vi "Initialize.vi"(8 "error in":errorcluster, 10 "parameters":variant, 11 "Sync Channel in":refnum<class "Synchronization Channel.lvclass">) -> (0 "error out":errorcluster, 2 "summary":T2[](array[typedef]), 3 "data value reference":T1)   [LabVIEW 2025, in "Synchronization.lvlib" / "Synchronization Channel.lvclass"]
doc: "This Vi initializes the data of a node its default state.\nThe object is not created inside of this ViI, beacuase it is created from a File depending on user selection.Copyright 2017 National Instruments Corporation\n\nLicensed under the Apache License, Version 2.0 (the \"License\"); you may not use this file except in compliance with the License. You may obtain a copy of the License at http://www.apache.org/licenses/LICENSE-2.0\nUnless required by applicable law or agreed to in writing, software distributed under the License is distributed on an \"AS IS\" BASIS, WITHOUT WARRANTIES OR CONDITIONS OF ANY KIND, either express or implied. See the License for the specific language governing permissions and limitations under the License."
uses:
  Synchronization Channel.lvclass
  Synchronization Channel.lvclass/Synchronization Channel.ctl
  Users/Public/Documents/Sandia National Labs/TSS Plugin/CEF.lvlibp/Node/CEF_Node.lvclass
  Synchronization Instrument/Synchronization Instrument.lvclass
  Synchronization configuration/Synchronization configuration.lvclass
  Synchronization Channel configuration/Synchronization Channel configuration.lvclass
  Users/Public/Documents/Sandia National Labs/TSS Plugin/Abstract Engine.lvlibp/Plugin/Abstract/Abstract Channel/Abstract Channel.lvclass
  Users/Public/Documents/Sandia National Labs/TSS Plugin/CEF.lvlibp/Node/NodeRef.ctl
  Users/Public/Documents/Sandia National Labs/TSS Plugin/CEF.lvlibp/Node/Summary.ctl
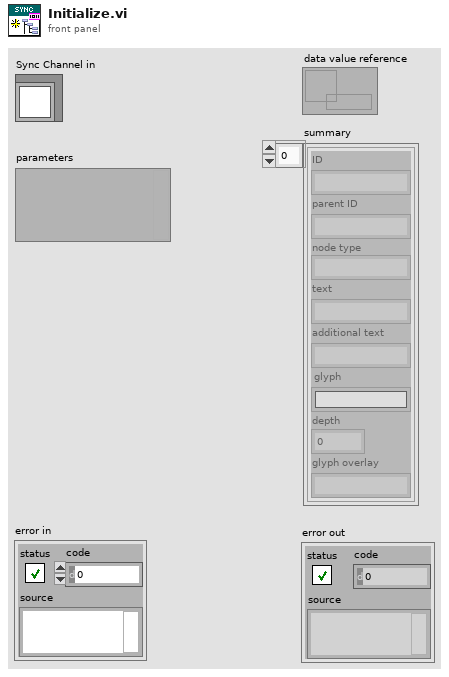
[diagram p1: front panel]
types:
  T1 = typedef "CEF.lvlibp/CEF_Node.lvclass/NodeRef.ctl" = refnum<data-value>
  T2 = typedef "CEF.lvlibp/CEF_Node.lvclass/Summary.ctl" = cluster{"ID":string, "parent ID":string, "node type":string, "text":string, "additional text":string, "glyph":string, "depth":i32, "glyph overlay":string}
  T3 = cluster{"Type":string, "Address":string, "SW Alias":string, "Description":string, "Enabled":bool}
  T4 = cluster{"Address":string, "SW Alias":string, "Enabled":bool, "Type":string, "Description":string}
  T5 = cluster{"ID":string, "parent ID":string, "node type":string, "text":string, "additional text":string, "glyph":string, "depth":i32, "glyph overlay":string}[]
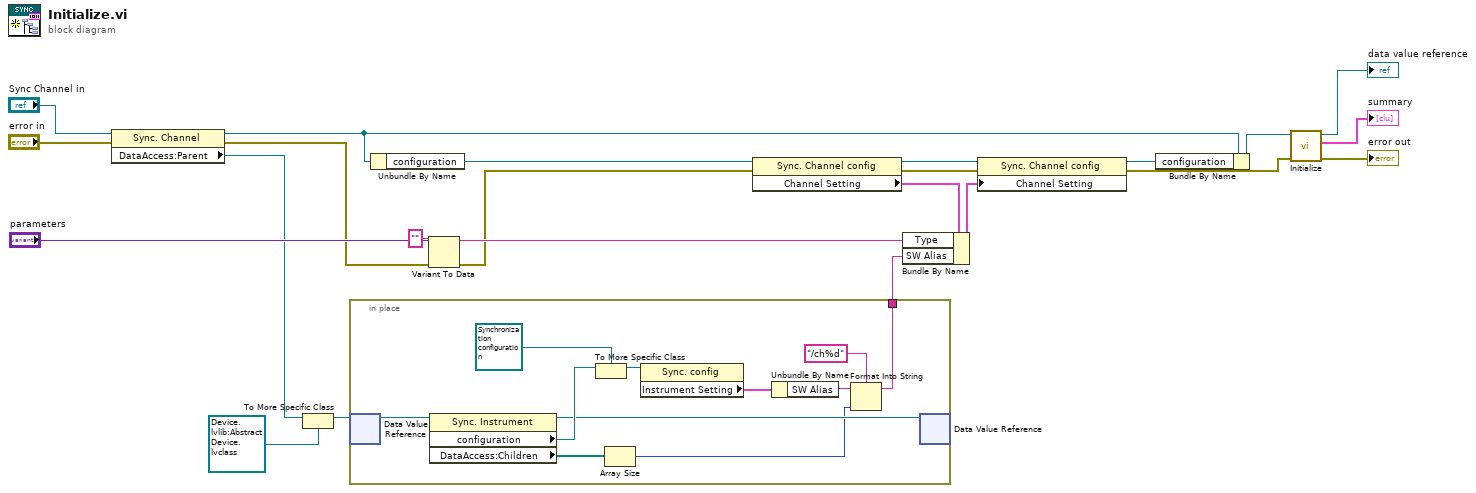
[diagram p0: block diagram]
diagram:
  n1 = property class="Sync. Channel"(reference="Sync Channel in", error in="error in") -> (reference out=w6:refnum<class "Synchronization Channel.lvclass">, error out=w9:errorcluster, "DataAccess:Parent"=w17:refnum<data-value>)
  n2 = To More Specific Class(target class=refnum<data-value> refnum ("data value reference"), reference=w17) -> (specific class reference=w18:refnum<data-value>)  [unwired: 1 in, 1 out]
  n3 = in-place {
    in-place-border: [w31] -> w10
    n4 = in-place-dvr #1(w18) -> (w30:refnum<class "Synchronization Instrument.lvclass">)  [unwired: 1 out]
    n5 = property class="Sync. Instrument"(reference=w30) -> (reference out=w26:refnum<class "Synchronization Instrument.lvclass">, "configuration"=w29:refnum<class "CEF_serializable configuration.lvclass">, "DataAccess:Children"=w28:refnum<data-value>[])  [unwired: 1 in, 1 out]
    n6 = To More Specific Class(target class=refnum<class "Synchronization configuration.lvclass"> refnum ("Device.lvlib:Device configuration.lvclass"), reference=w29) -> (specific class reference=w34:refnum<class "Synchronization configuration.lvclass">)  [unwired: 1 in, 1 out]
    n7 = Array Size(array=w28) -> (size(s)=w25:i32)
    n8 = property class="Sync. config"(reference=w34) -> ("Instrument Setting"=w24:T3)  [unwired: 1 in, 2 out]
    n9 = Unbundle By Name(w24) -> ("SW Alias"=w33:string)
    n10 = Format Into String(format string="/ch%d", initial string=w33, w25) -> (resulting string=w31:string)  [unwired: 1 in, 1 out]
    n11 = in-place-dvr #1(w26) -> ()  [unwired: 2 out]
  }
  n12 = Unbundle By Name(w6) -> ("configuration"=w16:refnum<class "Synchronization Channel configuration.lvclass">)
  n13 = Variant To Data(error in=w9, type="" ("Class"), Variant="parameters") -> (data=w11:string, error out=w5:errorcluster)
  n14 = property class="Sync. Channel config"(reference=w16, error in=w5) -> (reference out=w12:refnum<class "Synchronization Channel configuration.lvclass">, error out=w2:errorcluster, "Channel Setting"=w4:T4)
  n15 = Bundle By Name(cluster=w4, "Type"=w11, "SW Alias"=w10) -> (w3:T4)
  n16 = property class="Sync. Channel config"(reference=w12, error in=w2, "Channel Setting"=w3) -> (reference out=w14:refnum<class "Synchronization Channel configuration.lvclass">, error out=w8:errorcluster)
  n17 = Bundle By Name(cluster=w6, "configuration"=w14) -> (w15:refnum<class "Synchronization Channel.lvclass">)
  n18 = call-parent "Initialize.vi"("error in"=w8, "CEF_Serialize node in"=w15) -> ("error out"=→"error out":errorcluster, "summary"=→"summary":T5, "data value reference"=→"data value reference":refnum<data-value>)  [unwired: 7 in]
